vi "ArraysFunctions1.vi"() -> ()   [LabVIEW 2020]
panel:
  in  "dimension size":i32
  out "output array":i32[](array[numeric])
  out "size(s)":i32[](array[numeric])
  out "Array":i32[][](array[numeric])
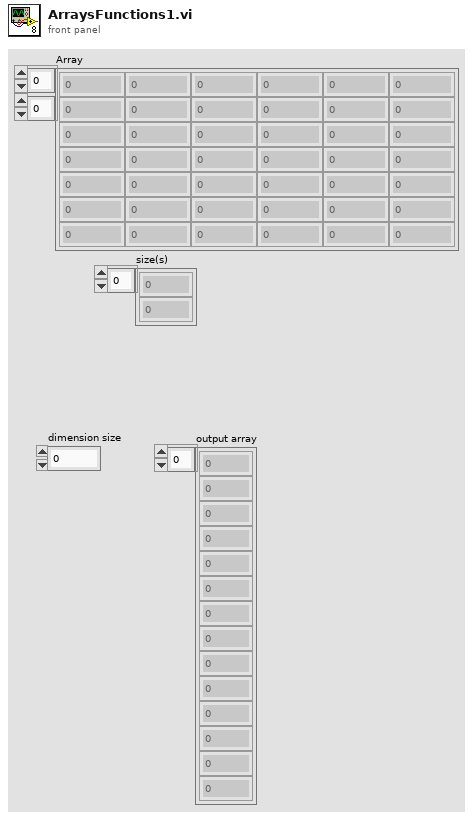
[diagram p1: front panel]
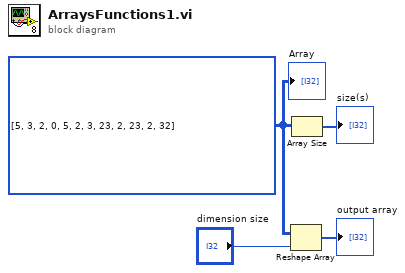
[diagram p0: block diagram]
diagram:
  w3 = i32[][] [[5, 3, 2], [0, 5, 2], [3, 23, 2], [23, 2, 32]]
  n1 = Reshape Array(w3, "dimension size") -> (→"output array":i32[])
  n2 = Array Size(array=w3) -> (size(s)=→"size(s)":i32[])
  "Array" <- w3
